vi "determine warnings VI.vi"() -> ()   [LabVIEW 2014]
panel:
  out "Warning?":bool
  out "Warnign Text":string
  in  "Min Temp":dbl
  in  "Max Temp":dbl
  in  "Current Temp":dbl
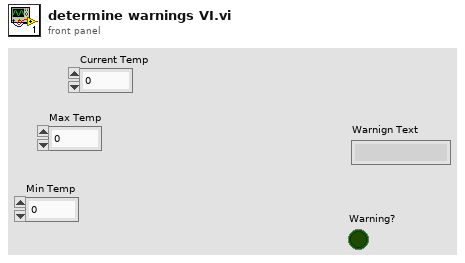
[diagram p1: front panel]
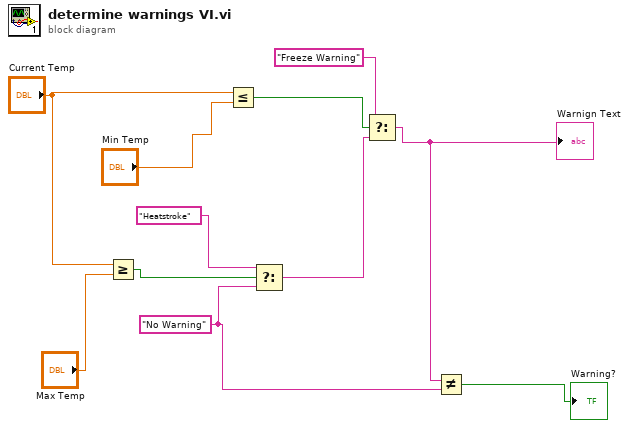
[diagram p0: block diagram]
diagram:
  w2 = "No Warning"
  n1 = Greater Or Equal?(x="Current Temp", y="Max Temp") -> (x >= y?=w7:bool)
  n2 = Less Or Equal?(x="Current Temp", y="Min Temp") -> (x <= y?=w8:bool)
  n3 = Select(t="Heatstroke", s=w7, f=w2) -> (s? t:f=w5:string)
  n4 = Select(t="Freeze Warning", s=w8, f=w5) -> (s? t:f=w3:string)
  "Warnign Text" <- w3
  n5 = Not Equal?(x=w3, y=w2) -> (x != y?=→"Warning?":bool)
